vi "I2C Thermocouple MCP9600.vi"() -> ()   [LabVIEW 2020, in "CTI-Scratchpad.lvlib"]
uses:
  CTI-Scratchpad.lvlib
  CTI/Identity.ctl
  CTI/CTI-Grove/Examples/Sourcecode/cti-drivers-lv-visa-simple/Examples/I2C/Thermocouple(MCP9600)/ThermocoupleType.ctl
  CTI/Error Reporting.ctl
  CTI/GPIO Number.ctl
  CTI/I2C Number.ctl
  CTI/Session/Session.lvclass
  CTI-Peripheral/Analog Input/Grove I2C Sensors/Thermocouple/Grove Thermocouple MCP9600.lvclass
  CTI/VisaComms/VisaComms.lvclass
  CTI/CTI.lvlib
panel:
  out "Thermometer":dbl(slide) scale=0.0..1000.0
  in  "Thermocouple Type":T1
  out "Temperature":dbl(graph)
  in  "Stop":bool
  out "loop":i32
  out "Identity":T2
  in  "Grove Connector":enum16{"I2C0", "I2C1"}(ring)
  out "error out":errorcluster
  in  "Port":refnum<visa-resource-name>="COM4"
  # "https://wiki.seeedstudio.com/Grove-I2C_Thermocouple_Amplifier-MCP9600/"
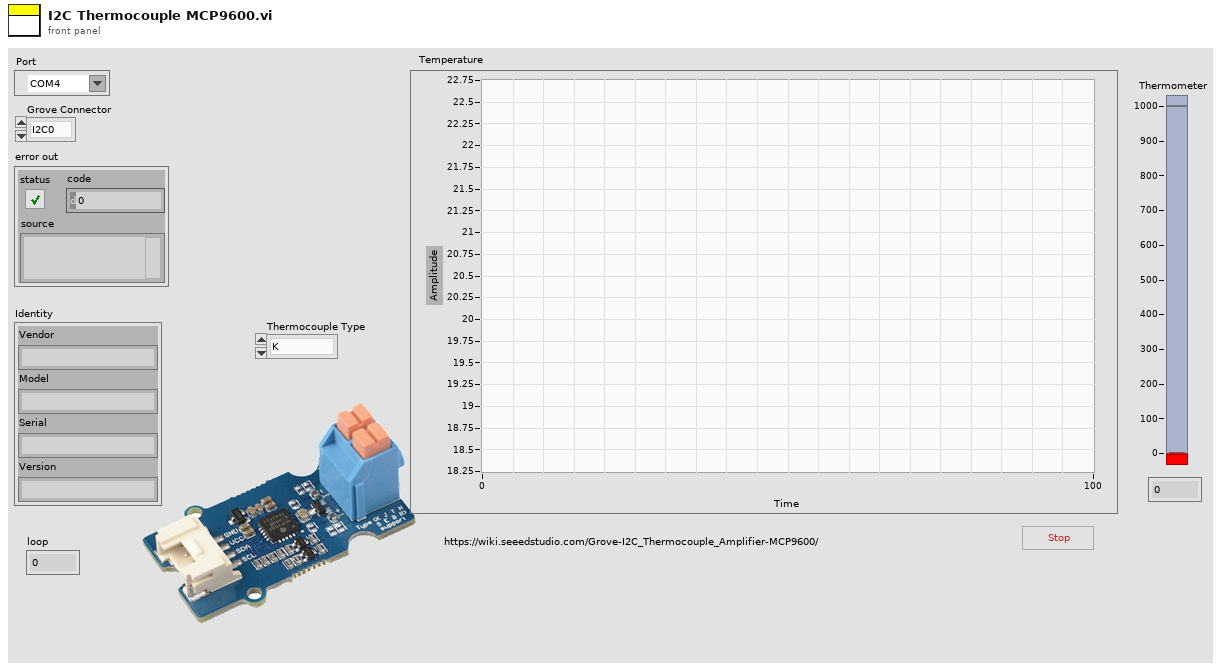
[diagram p1: front panel]
types:
  T1 = typedef "ThermocoupleType.ctl" = enum16{"K", "J", "T", "N", "S", "E", "B", "R"}
  T2 = typedef "CTI.lvlib/Identity.ctl" = cluster{"Vendor":string, "Model":string, "Serial":string, "Version":string}
  T3 = typedef "CTI.lvlib/Error Reporting.ctl" = enum16{"Minimal", "Moderate", "Full"}
  T4 = typedef "CTI.lvlib/I2C Number.ctl" = i8
  T5 = typedef "CTI.lvlib/GPIO Number.ctl" = i8
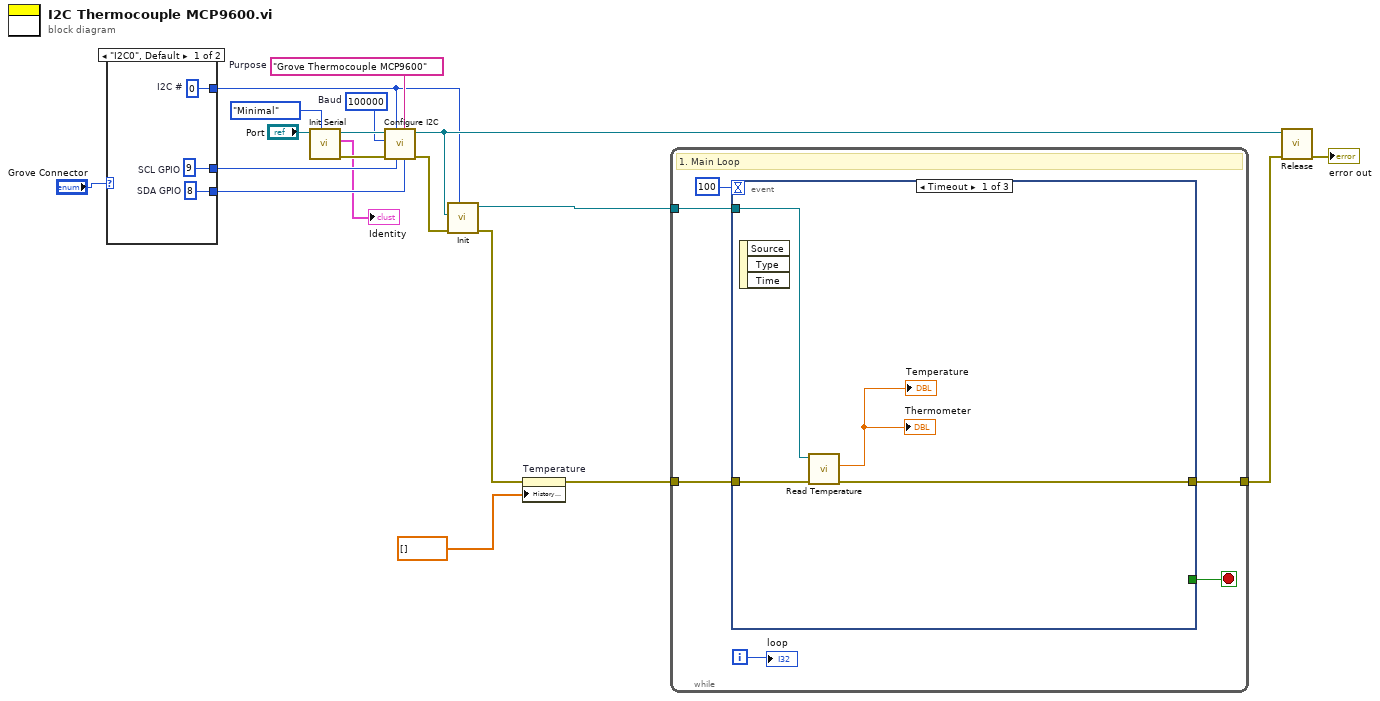
[diagram p0: block diagram]
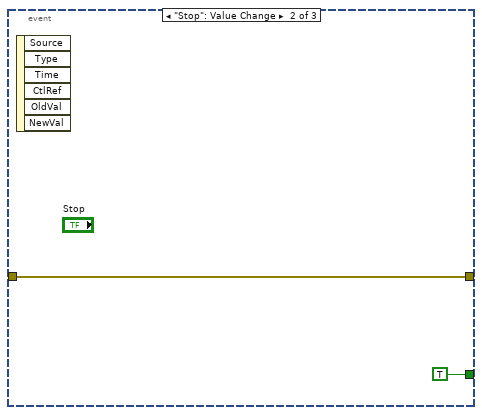
[diagram p2: hidden frame]
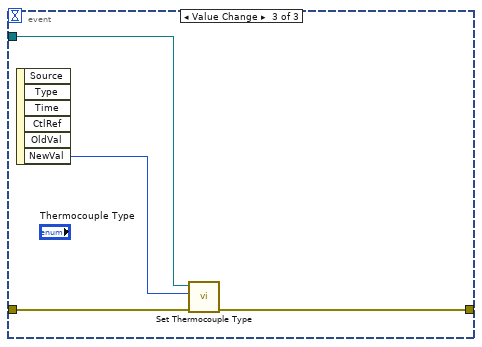
[diagram p3: hidden frame]
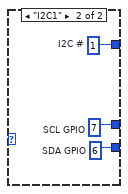
[diagram p4: hidden frame]
diagram:
  w14 = "Grove Thermocouple MCP9600"  # Purpose
  w15 = u32 100000  # Baud
  n1 = case shown="\"I2C0\", Default" "Grove Connector" {
    tunnel: [w22 w25] -> w10
    tunnel: [w21 w24] -> w9
    tunnel: [w20 w23] -> w8
    frame "I2C0", Default {
      w20 = T4 0  # I2C #
      w21 = T5 8  # SDA GPIO
      w22 = T5 9  # SCL GPIO
    }
    frame "I2C1" {
      w23 = T4 1  # I2C #
      w24 = T5 6  # SDA GPIO
      w25 = T5 7  # SCL GPIO
    }
  }
  n2 = call "Init Serial.vi"("Error Checking (Full)"=Error_Reporting."Minimal", "VISA resource name in"="Port") -> ("error out"=w16:errorcluster, "Identity"=→"Identity":T2, "Session"=w17:refnum<class "Session.lvclass">)  [unwired: 7 in]
  n3 = call "Configure I2C.vi"("SDA GPIO"=w9, "Purpose (\"I2C\")"=w14, "SCL GPIO"=w10, "I2C #"=w8, "error in (no error)"=w16, "Baud"=w15, "Session in"=w17) -> ("error out"=w13:errorcluster, "Session out"=w12:refnum<class "Session.lvclass">)  [unwired: 3 in]
  n4 = call "Init.vi"("I2C #"=w8, "error in (no error)"=w13, "Session In"=w12) -> ("error out"=w3:errorcluster, "Grove Thermocouple MCP9600"=w6:refnum<class "Grove Thermocouple MCP9600.lvclass">)  [unwired: 7 in]
  n5 = property on="Temperature" class="WFChart (strict)"(error in=w3, "History Data"=dbl[] []) -> (error out=w2:errorcluster)  [unwired: 1 in, 1 out]
  n6 = while {
    tunnel: w2 -> [w30]
    tunnel: w6 -> [w31]
    tunnel: [w28] -> w5
    i -> [w29]
    stop <- w26 stop-if-true
    # "1. Main Loop"
    n7 = event shown="[0] Timeout" {
      selector: _ -> [_ _ _]
      dyn-events: _ -> [_ _ _]
      timeout: 100 -> [_ _ _]
      tunnel: w31 -> [w34 _ w41]
      tunnel: w30 -> [w35 w36 w39]
      tunnel: [w33 w36 w38] -> w28
      tunnel: [_ TRUE _] -> w26
      event Timeout {
        n8 = event-data() -> ()  [unwired: 1 in, 3 out]
        n9 = call-dynamic "Read Temperature.vi"("error in (no error)"=w35, "Grove Thermocouple MCP9600 in"=w34) -> ("error out"=w33:errorcluster, "Temperature"=→"Temperature" →"Thermometer":dbl)  [unwired: 7 in, 1 out]
      }
      event "Stop": Value Change {
        n10 = event-data() -> ()  [unwired: 1 in, 6 out]
      }
      event Value Change {
        n11 = event-data() -> ("NewVal"=w40:T1)  [unwired: 1 in, 5 out]
        n12 = call-dynamic "Set Thermocouple Type.vi"("error in (no error)"=w39, "Thermocouple Type"=w40, "Grove Thermocouple MCP9600 in"=w41) -> ("error out"=w38:errorcluster)  [unwired: 7 in, 1 out]
      }
    }
    "loop" <- w29
  }
  n13 = call-dynamic "Release.vi"("error in (no error)"=w5, "Session in"=w12) -> ("error out"=→"error out":errorcluster)  [unwired: 9 in]
